vi "sin-cos-generatorA.vi"(2 "Time":dbl format="%.2f", 3 "Phase":dbl format="%.2f", 4 "Frequency":dbl format="%.2f") -> (0 "cos":dbl format="%.2f", 1 "sin":dbl format="%.2f")   [LabVIEW 2013]
uses:
  <vilib>/ptbypt/NI_PtbyPt.lvlib
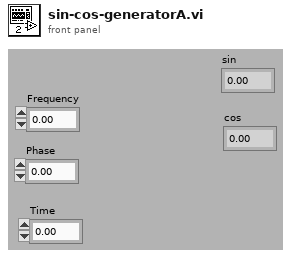
[diagram p1: front panel]
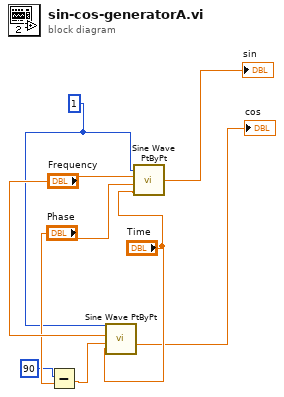
[diagram p0: block diagram]
diagram:
  w3 = 1
  n1 = Subtract(x=90, y="Phase") -> (x-y=w5:dbl)
  n2 = call <vilib>:"Sine Wave PtByPt.vi"("time"="Time", "phase"=w5, "frequency"="Frequency", "amplitude"=w3) -> ("sine wave"=→"cos":dbl)
  n3 = call <vilib>:"Sine Wave PtByPt.vi"("time"="Time", "phase"="Phase", "frequency"="Frequency", "amplitude"=w3) -> ("sine wave"=→"sin":dbl)
